vi "filter_frequency_imp_test_v3.vi"() -> ()   [LabVIEW 2014]
uses:
  <vilib>/rvi/Analysis/host/Butterworth/config/Butterworth Filter Order.ctl
  <vilib>/rvi/Analysis/host/Butterworth/config/Butterworth Filter Type.ctl
  <vilib>/FPGAPlugInAG/cRIO-9039/niLvFpga_Open_cRIO-9039.vi
  <vilib>/rvi/interface/common/dynamic/niFpgaDynamicAddResources.vi
  <vilib>/rvi/Analysis/host/Butterworth/config/BwScaledCoefficients.vi
  <vilib>/Utility/error.llb/Error Cluster From Error Code.vi
  <vilib>/rvi/errors/niLvFpgaAdjustHostInterfaceError.vi
  <vilib>/FPGAPlugInAG/Dynamic/niLvFpga_Close_Dynamic.vi
  <vilib>/rvi/interface/nirviOpenFPGA/nirviOpenFPGA.xnode
  FPGA Bitfiles/test0304_FPGATarget_imptestv3_S4g9B0kYVuk.lvbitx
  imp_test_v3.vi
  <vilib>/rvi/Analysis/host/Butterworth/XNode/ButterworthCoefficients.xnode
  <vilib>/rvi/interface/nirviReadWriteControl/nirviReadWriteControl.xnode
  <vilib>/rvi/interface/nirviCloseFPGA/nirviCloseFPGA.xnode
  <vilib>/rvi/Analysis/host/Public/NI_FpgaMspHost.lvlib
  NiFpgaLv.dll
  <vilib>/rvi/interface/Simulation/niFpgaSimulationCallBeginRW.vi
panel:
  in  "sr_Strain(mean) (S/s)":dbl=50000.0
  in  "fcu_Strain(mean) (Hz)":dbl=1000.0
  in  "sr_ft_d (S/s)":dbl=50000.0
  in  "fcu_ft_d (Hz)":dbl=1000.0
  in  "sr_D_dd (S/s)":dbl=50000.0
  in  "fcu_D_dd (Hz)":dbl=1000.0
  in  "sr_dF_PID (S/s)":dbl=50000.0
  in  "fcu_dF_PID (Hz)":dbl=1000.0
  in  "sr_Strain (S/s)":dbl=50000.0
  in  "fcu_Strain (Hz)":dbl=1000.0
  in  "stop":bool
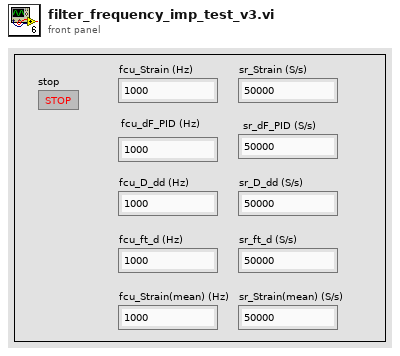
[diagram p1: front panel]
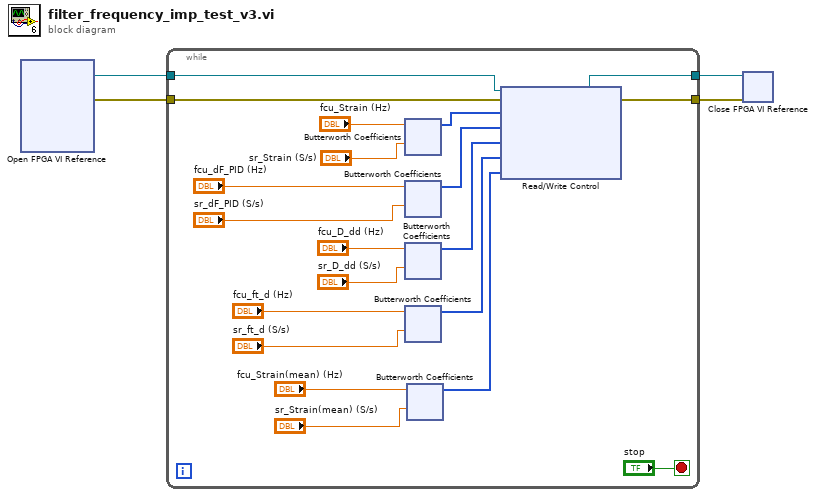
[diagram p0: block diagram]
diagram:
  n1 = xnode "Open FPGA VI Reference"() -> ("FPGA VI Reference Out"=w4:refnum<k20>, "error out"=w3:errorcluster)  [unwired: 2 in]
  n2 = while {
    tunnel: w4 -> [w23]
    tunnel: w3 -> [w22]
    tunnel: [w21] -> w2
    tunnel: [w20] -> w1
    stop <- "stop" stop-if-true
    n3 = xnode "Butterworth Coefficients"("cutoff frequency (Hz)"="fcu_Strain (Hz)", "sample rate (S/s)"="sr_Strain (S/s)") -> ("scaled coefficients"=w19:i32[])  [unwired: 1 in, 1 out]
    n4 = xnode "Butterworth Coefficients"("cutoff frequency (Hz)"="fcu_dF_PID (Hz)", "sample rate (S/s)"="sr_dF_PID (S/s)") -> ("scaled coefficients"=w18:i32[])  [unwired: 1 in, 1 out]
    n5 = xnode "Butterworth Coefficients"("cutoff frequency (Hz)"="fcu_D_dd (Hz)", "sample rate (S/s)"="sr_D_dd (S/s)") -> ("scaled coefficients"=w17:i32[])  [unwired: 1 in, 1 out]
    n6 = xnode "Butterworth Coefficients"("cutoff frequency (Hz)"="fcu_ft_d (Hz)", "sample rate (S/s)"="sr_ft_d (S/s)") -> ("scaled coefficients"=w16:i32[])  [unwired: 1 in, 1 out]
    n7 = xnode "Butterworth Coefficients"("cutoff frequency (Hz)"="fcu_Strain(mean) (Hz)", "sample rate (S/s)"="sr_Strain(mean) (S/s)") -> ("scaled coefficients"=w7:i32[])  [unwired: 1 in, 1 out]
    n8 = xnode "Read/Write Control"("FPGA VI Reference In"=w23, "error in"=w22, "Strain filter coeff."=w19, "dF_PID coeff."=w18, "D_dd coeff."=w17, "ft_d coeff."=w16, "Strain mean coeff."=w7) -> ("FPGA VI Reference Out"=w21:refnum<k20>, "error out"=w20:errorcluster)
  }
  n9 = xnode "Close FPGA VI Reference"("FPGA VI Reference In"=w2, "error in"=w1) -> ()  [unwired: 1 out]
